vi "Setup Motors.vi"   [LabVIEW 2014]
uses:
  <vilib>/Rock Robotics/SystemInterfaces/DIO/FPGA_DIOPWMChannel.ctl
  <vilib>/Rock Robotics/SystemInterfaces/Typedef/FPGA_TypedefDigitalModule.ctl
  <vilib>/Rock Robotics/WPI/Joystick/WPI_JoystickDeviceEnum.ctl
  <vilib>/Rock Robotics/SystemInterfaces/Typedef/FPGA_TypedefAnalogModule.ctl
  <vilib>/Rock Robotics/SystemInterfaces/AI/FPGA_AIChannel.ctl
  <vilib>/Rock Robotics/WPI/Solenoid/WPI_SolenoidChannel.ctl
  <vilib>/Rock Robotics/SystemInterfaces/AI/FPGA_AIGyroChannel.ctl
  <vilib>/Rock Robotics/SystemInterfaces/Typedef/FPGA_TypedefAnalogModuleForGyro.ctl
  <vilib>/Rock Robotics/SystemInterfaces/DIO/FPGA_DIOChannel.ctl
  <vilib>/Rock Robotics/WPI/SafetyOutput/WPI_SafetyOutputConfigMenu.ctl
  <vilib>/Rock Robotics/WPI/MotorControl/WPI_MotorControlOpen Talon.vi
  <vilib>/Rock Robotics/WPI/Solenoid/WPI_SolenoidOpenSingle.vi
  <vilib>/Rock Robotics/WPI/Switch/WPI_SwitchOpenLimit.vi
  <vilib>/Rock Robotics/WPI/Counter/WPI_CounterDigitalInputToDigitalSource.vi
  Global Variables.vi
types:
  T1 = typedef "FPGA_DIOChannel.ctl" = enum8{"DIO 0", "DIO 1", "DIO 2", "DIO 3", "DIO 4", "DIO 5", "DIO 6", "DIO 7", "DIO 8", "DIO 9", "DIO MXP 0", "DIO MXP 1", "DIO MXP 2", "DIO MXP 3", "DIO MXP 4", "DIO MXP 5", "DIO MXP 6", "DIO MXP 7", "DIO MXP 8", "DIO MXP 9", "DIO MXP 10", "DIO MXP 11", "DIO MXP 12", "DIO MXP 13", "DIO MXP 14", "DIO MXP 15", "Invalid"}
  T2 = typedef "WPI_SafetyOutputConfigMenu.ctl" = enum16{"Enable", "Disable"}
  T3 = typedef "FPGA_DIOPWMChannel.ctl" = enum8{"PWM 0", "PWM 1", "PWM 2", "PWM 3", "PWM 4", "PWM 5", "PWM 6", "PWM 7", "PWM 8", "PWM 9", "PWM MXP 0", "PWM MXP 1", "PWM MXP 2", "PWM MXP 3", "PWM MXP 4", "PWM MXP 5", "PWM MXP 6", "PWM MXP 7", "PWM MXP 8", "PWM MXP 9", "Invalid"}
  T4 = typedef "FPGA_TypedefDigitalModule.ctl" = enum16{"Controller 1"}
  T5 = typedef "FPGA_TypedefAnalogModuleForGyro.ctl" = enum16{"Controller 1"}
  T6 = typedef "FPGA_AIGyroChannel.ctl" = enum8{"AI 0", "AI 1", "Invalid"}
  T7 = typedef "WPI_SolenoidChannel.ctl" = enum8{"Solenoid 0", "Solenoid 1", "Solenoid 2", "Solenoid 3", "Solenoid 4", "Solenoid 5", "Solenoid 6", "Solenoid 7", "Invalid"}
  T8 = typedef "FPGA_AIChannel.ctl" = enum8{"AI 0", "AI 1", "AI 2", "AI 3", "AI MXP 0", "AI MXP 1", "AI MXP 2", "AI MXP 3", "Invalid"}
  T9 = typedef "FPGA_TypedefAnalogModule.ctl" = enum16{"Controller 1"}
  T10 = typedef "WPI_JoystickDeviceEnum.ctl" = enum16{"USB 0", "USB 1", "USB 2", "USB 3", "USB 4", "USB 5"}
  T11 = typedef "WPI_MotorControlDeviceRef.ctl" = cluster{"DeviceStatus":errorcluster, "Type":T12, "PWM":cluster{"Controller":T4, "PWM Channel":T3, "DeadBand":T13}, "CAN":cluster{"Device Number":u8, "Control Mode":T14, "Semaphore":T15, "Max Vout":dbl, "TalonSRX Control Mode":T16}, "Invert":bool, "TransformRef":T17, "InvTransformRef":T17}
  T12 = typedef "WPI_MotorControlType.ctl" = enum16{"PWM", "CAN", "CANTalonSRX"}
  T13 = typedef "WPI_PWMDeadband.ctl" = cluster{"Name":string, "maxPositivePwm":i32, "minPositivePwm":i32, "centerPwm":i32, "maxNegativePwm":i32, "minNegativePwm":i32, "angularRange":u16}
  T14 = typedef "WPI_CANJaguar_ControlMode.ctl" = enum8{"Percent VBus", "Current", "Speed", "Position", "Voltage"}
  T15 = typedef "Semaphore RefNum" = refnum<k1>
  T16 = typedef "WPI_CANTalonSRX_APIControlMode.ctl" = enum8{"Percent VBus", "Speed", "Position", "Slave", "Unchanged / Invalid"}
  T17 = typedef "WPI_PWMTransform_ConPane.ctl" = refnum<vi>
  T18 = typedef "WPI_GyroDevRef.ctl" = cluster{"DevStatus":errorcluster, "Analog Module":T9, "Analog Channel":T8, "Offset":dbl, "Gain (VoltsPerDegree/Second)":dbl}
  T19 = typedef "WPI_SolenoidDevRef.ctl" = cluster{"DevStatus":errorcluster, "Pneumatics Control Module":u8, "Forward Solenoid Channel":T7, "Reverse Solenoid Channel":T7}
  T20 = typedef "WPI_SwitchDevRef.ctl" = cluster{"DevStatus":errorcluster, "DIO Channel":T1, "Controller":T4, "CntIndex":T21, "Normally Closed":bool}
  T21 = typedef "FPGA_CounterCtrSystemIndex.ctl" = enum8{"Ctr 0", "Ctr 1", "Ctr 2", "Ctr 3", "Ctr 4", "Ctr 5", "Ctr 6", "Ctr 7", "Invalid"}
  T22 = typedef "WPI_DigitalInputDevRef.ctl" = cluster{"DevStatus":errorcluster, "DIO Channel":T1, "Controller":T4}
  T23 = typedef "FPGA_CounterEncoderSourceConvertionLVSourceType.ctl" = cluster{"DevStatus":errorcluster, "AnalogTriggerMode?":bool, "DigitalMode":cluster{"Controller":T4, "DIO Channel":T24}, "AnalogTriggerMode":cluster{"AnalogTriggerIndex":T25, "OutputType":T26}}
  T24 = typedef "FPGA_DIODigitalSourceChannel.ctl" = enum8{"DIO 0", "DIO 1", "DIO 2", "DIO 3", "DIO 4", "DIO 5", "DIO 6", "DIO 7", "DIO 8", "DIO 9", "DIO MXP 0", "DIO MXP 1", "DIO MXP 2", "DIO MXP 3", "DIO MXP 4", "DIO MXP 5", "DIO MXP 6", "DIO MXP 7", "DIO MXP 8", "DIO MXP 9", "DIO MXP 10", "DIO MXP 11", "DIO MXP 12", "DIO MXP 13", "DIO MXP 14", "DIO MXP 15", "Disabled"}
  T25 = typedef "FPGA_AnalogTriggerIndex.ctl" = enum8{"Trig 0", "Trig 1", "Trig 2", "Trig 3", "Trig 4", "Trig 5", "Trig 6", "Trig 7", "Invalid"}
  T26 = typedef "FPGA_AnalogTriggerOutType.ctl" = enum16{"InWindow", "TriggerState", "Rising", "Falling"}
  T27 = typedef "WPI_AnalogChannelDevRef.ctl" = cluster{"DevStatus":errorcluster, "Controller":T9, "Analog Channel":T8}
  T28 = typedef "WPI_EncoderDevRef.ctl" = cluster{"DevStatus":errorcluster, "EncoderIndex":T29, "CounterIndex":T21, "DistancePerCount":dbl, "Decoding Type":T30}
  T29 = typedef "FPGA_EncoderIdx.ctl" = enum8{"Enc 0", "Enc 1", "Enc 2", "Enc 3", "Enc 4", "Enc 5", "Enc 6", "Enc 7", "Invalid"}
  T30 = typedef "WPI_EncoderType.ctl" = enum16{"1x", "2x", "4x"}
  T31 = typedef "WPI_JoystickDevRef.ctl" = cluster{"Device":T10}
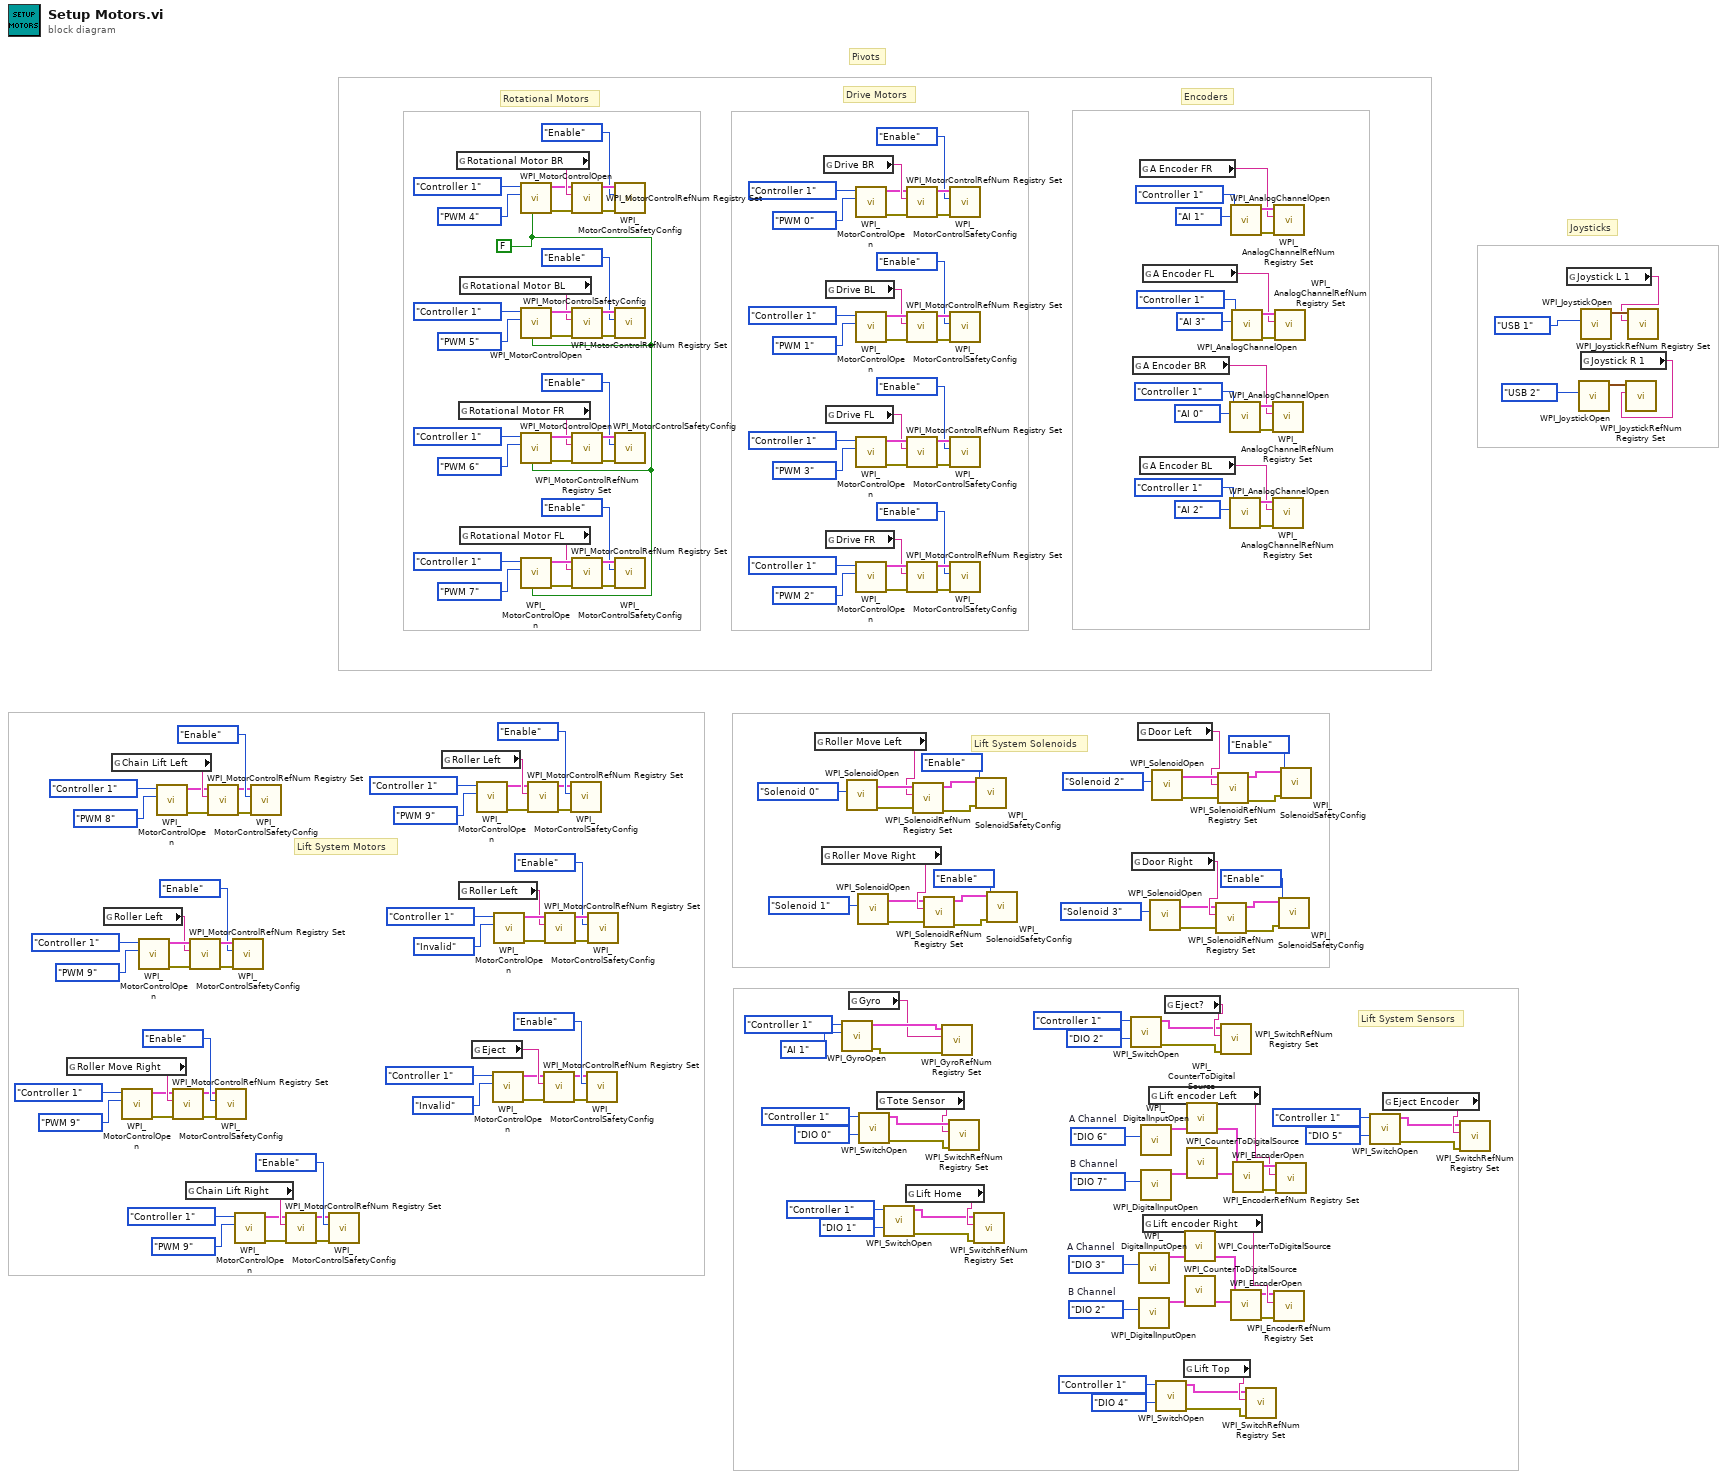
[diagram p0: block diagram]
diagram:
  w1 = FPGA_DIOChannel."DIO 2"  # B Channel
  w2 = FPGA_DIOChannel."DIO 3"  # A Channel
  w18 = FALSE ("Invert")
  w27 = FPGA_DIOChannel."DIO 7"  # B Channel
  w26 = FPGA_DIOChannel."DIO 6"  # A Channel
  # "Lift System Sensors"
  # "Lift System Solenoids"
  # "Lift System Motors"
  # "Encoders"
  # "Joysticks"
  # "Pivots"
  # "Rotational Motors"
  # "Drive Motors"
  n1 = global read "Global Variables.vi" "Roller Move Right"() -> (w116:string)
  n2 = global read "Global Variables.vi" "Roller Left"() -> (w119:string)
  n3 = global read "Global Variables.vi" "Chain Lift Left"() -> (w132:string)
  n4 = call-poly <vilib>:"WPI_MotorControlOpen.vi"("PWM Channel"=FPGA_DIOPWMChannel."PWM 9", "Controller"=FPGA_TypedefDigitalModule."Controller 1") -> ("error out"=w111:errorcluster, "MotorControlDeviceRef"=w110:T11)  [unwired: 8 in]
  n5 = call-poly <vilib>:"WPI_MotorControlOpen.vi"("PWM Channel"=FPGA_DIOPWMChannel."PWM 9", "Controller"=FPGA_TypedefDigitalModule."Controller 1") -> ("error out"=w124:errorcluster, "MotorControlDeviceRef"=w125:T11)  [unwired: 8 in]
  n6 = call-poly <vilib>:"WPI_MotorControlOpen.vi"("PWM Channel"=FPGA_DIOPWMChannel."PWM 8", "Controller"=FPGA_TypedefDigitalModule."Controller 1") -> ("error out"=w127:errorcluster, "MotorControlDeviceRef"=w126:T11)  [unwired: 8 in]
  n7 = call <vilib>:"WPI_MotorControlRefNum Registry Set.vi"("error in (no error)"=w111, "refnum name"=w116, "MotorControlDevRef"=w110) -> ("error out"=w113:errorcluster, "MotorControlDevRef"=w112:T11)  [unwired: 7 in]
  n8 = global read "Global Variables.vi" "Chain Lift Right"() -> (w16:string)
  n9 = call <vilib>:"WPI_MotorControlRefNum Registry Set.vi"("error in (no error)"=w124, "refnum name"=w119, "MotorControlDevRef"=w125) -> ("error out"=w122:errorcluster, "MotorControlDevRef"=w123:T11)  [unwired: 7 in]
  n10 = call <vilib>:"WPI_MotorControlRefNum Registry Set.vi"("error in (no error)"=w127, "refnum name"=w132, "MotorControlDevRef"=w126) -> ("error out"=w129:errorcluster, "MotorControlDevRef"=w128:T11)  [unwired: 7 in]
  n11 = call <vilib>:"WPI_MotorControlSafetyConfig.vi"("error in (no error)"=w113, "mode"=WPI_SafetyOutputConfigMenu."Enable", "MotorControlDevRef"=w112) -> ()  [unwired: 7 in, 2 out]
  n12 = call <vilib>:"WPI_MotorControlSafetyConfig.vi"("error in (no error)"=w122, "mode"=WPI_SafetyOutputConfigMenu."Enable", "MotorControlDevRef"=w123) -> ()  [unwired: 7 in, 2 out]
  n13 = call-poly <vilib>:"WPI_MotorControlOpen.vi"("PWM Channel"=FPGA_DIOPWMChannel."PWM 9", "Controller"=FPGA_TypedefDigitalModule."Controller 1") -> ("error out"=w11:errorcluster, "MotorControlDeviceRef"=w10:T11)  [unwired: 8 in]
  n14 = call <vilib>:"WPI_MotorControlSafetyConfig.vi"("error in (no error)"=w129, "mode"=WPI_SafetyOutputConfigMenu."Enable", "MotorControlDevRef"=w128) -> ()  [unwired: 7 in, 2 out]
  n15 = call <vilib>:"WPI_MotorControlRefNum Registry Set.vi"("error in (no error)"=w11, "refnum name"=w16, "MotorControlDevRef"=w10) -> ("error out"=w13:errorcluster, "MotorControlDevRef"=w12:T11)  [unwired: 7 in]
  n16 = call <vilib>:"WPI_MotorControlSafetyConfig.vi"("error in (no error)"=w13, "mode"=WPI_SafetyOutputConfigMenu."Enable", "MotorControlDevRef"=w12) -> ()  [unwired: 7 in, 2 out]
  n17 = global read "Global Variables.vi" "Roller Left"() -> (w108:string)
  n18 = global read "Global Variables.vi" "Rotational Motor BR"() -> (w186:string)
  n19 = global read "Global Variables.vi" "Rotational Motor FR"() -> (w160:string)
  n20 = global read "Global Variables.vi" "Roller Left"() -> (w95:string)
  n21 = global read "Global Variables.vi" "Rotational Motor BL"() -> (w161:string)
  n22 = global read "Global Variables.vi" "Rotational Motor FL"() -> (w159:string)
  n23 = global read "Global Variables.vi" "Eject"() -> (w92:string)
  n24 = call-poly <vilib>:"WPI_MotorControlOpen.vi"("PWM Channel"=FPGA_DIOPWMChannel."PWM 9", "Controller"=FPGA_TypedefDigitalModule."Controller 1") -> ("error out"=w103:errorcluster, "MotorControlDeviceRef"=w102:T11)  [unwired: 8 in]
  n25 = call-poly <vilib>:"WPI_MotorControlOpen.vi"("PWM Channel"=FPGA_DIOPWMChannel."Invalid", "Controller"=FPGA_TypedefDigitalModule."Controller 1") -> ("error out"=w87:errorcluster, "MotorControlDeviceRef"=w86:T11)  [unwired: 8 in]
  n26 = call-poly <vilib>:"WPI_MotorControlOpen.vi"("PWM Channel"=FPGA_DIOPWMChannel."Invalid", "Controller"=FPGA_TypedefDigitalModule."Controller 1") -> ("error out"=w100:errorcluster, "MotorControlDeviceRef"=w101:T11)  [unwired: 8 in]
  n27 = call-poly <vilib>:"WPI_MotorControlOpen.vi"("Invert"=w18, "PWM Channel"=FPGA_DIOPWMChannel."PWM 4", "Controller"=FPGA_TypedefDigitalModule."Controller 1") -> ("error out"=w184:errorcluster, "MotorControlDeviceRef"=w185:T11)  [unwired: 7 in]
  n28 = call-poly <vilib>:"WPI_MotorControlOpen.vi"("Invert"=w18, "PWM Channel"=FPGA_DIOPWMChannel."PWM 5", "Controller"=FPGA_TypedefDigitalModule."Controller 1") -> ("error out"=w178:errorcluster, "MotorControlDeviceRef"=w179:T11)  [unwired: 7 in]
  n29 = call-poly <vilib>:"WPI_MotorControlOpen.vi"("Invert"=w18, "PWM Channel"=FPGA_DIOPWMChannel."PWM 6", "Controller"=FPGA_TypedefDigitalModule."Controller 1") -> ("error out"=w172:errorcluster, "MotorControlDeviceRef"=w173:T11)  [unwired: 7 in]
  n30 = call-poly <vilib>:"WPI_MotorControlOpen.vi"("Invert"=w18, "PWM Channel"=FPGA_DIOPWMChannel."PWM 7", "Controller"=FPGA_TypedefDigitalModule."Controller 1") -> ("error out"=w166:errorcluster, "MotorControlDeviceRef"=w167:T11)  [unwired: 7 in]
  n31 = call <vilib>:"WPI_MotorControlRefNum Registry Set.vi"("error in (no error)"=w103, "refnum name"=w108, "MotorControlDevRef"=w102) -> ("error out"=w105:errorcluster, "MotorControlDevRef"=w104:T11)  [unwired: 7 in]
  n32 = call <vilib>:"WPI_MotorControlRefNum Registry Set.vi"("error in (no error)"=w87, "refnum name"=w92, "MotorControlDevRef"=w86) -> ("error out"=w89:errorcluster, "MotorControlDevRef"=w88:T11)  [unwired: 7 in]
  n33 = call <vilib>:"WPI_MotorControlRefNum Registry Set.vi"("error in (no error)"=w100, "refnum name"=w95, "MotorControlDevRef"=w101) -> ("error out"=w98:errorcluster, "MotorControlDevRef"=w99:T11)  [unwired: 7 in]
  n34 = call <vilib>:"WPI_MotorControlSafetyConfig.vi"("error in (no error)"=w105, "mode"=WPI_SafetyOutputConfigMenu."Enable", "MotorControlDevRef"=w104) -> ()  [unwired: 7 in, 2 out]
  n35 = call <vilib>:"WPI_MotorControlRefNum Registry Set.vi"("error in (no error)"=w184, "refnum name"=w186, "MotorControlDevRef"=w185) -> ("error out"=w182:errorcluster, "MotorControlDevRef"=w183:T11)  [unwired: 7 in]
  n36 = call <vilib>:"WPI_MotorControlRefNum Registry Set.vi"("error in (no error)"=w178, "refnum name"=w161, "MotorControlDevRef"=w179) -> ("error out"=w176:errorcluster, "MotorControlDevRef"=w177:T11)  [unwired: 7 in]
  n37 = call <vilib>:"WPI_MotorControlRefNum Registry Set.vi"("error in (no error)"=w172, "refnum name"=w160, "MotorControlDevRef"=w173) -> ("error out"=w170:errorcluster, "MotorControlDevRef"=w171:T11)  [unwired: 7 in]
  n38 = call <vilib>:"WPI_MotorControlRefNum Registry Set.vi"("error in (no error)"=w166, "refnum name"=w159, "MotorControlDevRef"=w167) -> ("error out"=w164:errorcluster, "MotorControlDevRef"=w165:T11)  [unwired: 7 in]
  n39 = call <vilib>:"WPI_MotorControlSafetyConfig.vi"("error in (no error)"=w89, "mode"=WPI_SafetyOutputConfigMenu."Enable", "MotorControlDevRef"=w88) -> ()  [unwired: 7 in, 2 out]
  n40 = call <vilib>:"WPI_MotorControlSafetyConfig.vi"("error in (no error)"=w98, "mode"=WPI_SafetyOutputConfigMenu."Enable", "MotorControlDevRef"=w99) -> ()  [unwired: 7 in, 2 out]
  n41 = call <vilib>:"WPI_MotorControlSafetyConfig.vi"("error in (no error)"=w182, "mode"=WPI_SafetyOutputConfigMenu."Enable", "MotorControlDevRef"=w183) -> ()  [unwired: 7 in, 2 out]
  n42 = call <vilib>:"WPI_MotorControlSafetyConfig.vi"("error in (no error)"=w176, "mode"=WPI_SafetyOutputConfigMenu."Enable", "MotorControlDevRef"=w177) -> ()  [unwired: 7 in, 2 out]
  n43 = call <vilib>:"WPI_MotorControlSafetyConfig.vi"("error in (no error)"=w170, "mode"=WPI_SafetyOutputConfigMenu."Enable", "MotorControlDevRef"=w171) -> ()  [unwired: 7 in, 2 out]
  n44 = call <vilib>:"WPI_MotorControlSafetyConfig.vi"("error in (no error)"=w164, "mode"=WPI_SafetyOutputConfigMenu."Enable", "MotorControlDevRef"=w165) -> ()  [unwired: 7 in, 2 out]
  n45 = global read "Global Variables.vi" "Roller Move Left"() -> (w80:string)
  n46 = global read "Global Variables.vi" "Roller Move Right"() -> (w79:string)
  n47 = global read "Global Variables.vi" "Drive BR"() -> (w223:string)
  n48 = global read "Global Variables.vi" "Drive BL"() -> (w198:string)
  n49 = global read "Global Variables.vi" "Drive FL"() -> (w197:string)
  n50 = global read "Global Variables.vi" "Drive FR"() -> (w196:string)
  n51 = call <vilib>:"WPI_GyroOpen.vi"("Analog Channel"=FPGA_AIGyroChannel."AI 1", "Controller"=FPGA_TypedefAnalogModuleForGyro."Controller 1") -> ("error out"=w60:errorcluster, "GyroDevRef"=w61:T18)  [unwired: 7 in, 1 out]
  n52 = call-poly <vilib>:"WPI_SolenoidOpen.vi"("Solenoid Channel"=WPI_SolenoidChannel."Solenoid 0") -> ("error out"=w82:errorcluster, "SolenoidDevRef"=w83:T19)  [unwired: 9 in]
  n53 = global read "Global Variables.vi" "Gyro"() -> (w57:string)
  n54 = call-poly <vilib>:"WPI_MotorControlOpen.vi"("PWM Channel"=FPGA_DIOPWMChannel."PWM 0", "Controller"=FPGA_TypedefDigitalModule."Controller 1") -> ("error out"=w221:errorcluster, "MotorControlDeviceRef"=w222:T11)  [unwired: 8 in]
  n55 = call-poly <vilib>:"WPI_MotorControlOpen.vi"("PWM Channel"=FPGA_DIOPWMChannel."PWM 1", "Controller"=FPGA_TypedefDigitalModule."Controller 1") -> ("error out"=w215:errorcluster, "MotorControlDeviceRef"=w216:T11)  [unwired: 8 in]
  n56 = call-poly <vilib>:"WPI_MotorControlOpen.vi"("PWM Channel"=FPGA_DIOPWMChannel."PWM 3", "Controller"=FPGA_TypedefDigitalModule."Controller 1") -> ("error out"=w209:errorcluster, "MotorControlDeviceRef"=w210:T11)  [unwired: 8 in]
  n57 = call-poly <vilib>:"WPI_MotorControlOpen.vi"("PWM Channel"=FPGA_DIOPWMChannel."PWM 2", "Controller"=FPGA_TypedefDigitalModule."Controller 1") -> ("error out"=w203:errorcluster, "MotorControlDeviceRef"=w204:T11)  [unwired: 8 in]
  n58 = call-poly <vilib>:"WPI_SolenoidOpen.vi"("Solenoid Channel"=WPI_SolenoidChannel."Solenoid 1") -> ("error out"=w77:errorcluster, "SolenoidDevRef"=w76:T19)  [unwired: 9 in]
  n59 = call-poly <vilib>:"WPI_SwitchOpen.vi"("DIO Channel"=FPGA_DIOChannel."DIO 0", "Controller"=FPGA_TypedefDigitalModule."Controller 1") -> ("error out"=w55:errorcluster, "SwitchDevRef"=w56:T20)  [unwired: 8 in]
  n60 = global read "Global Variables.vi" "Tote Sensor"() -> (w52:string)
  n61 = call-poly <vilib>:"WPI_SwitchOpen.vi"("DIO Channel"=FPGA_DIOChannel."DIO 1", "Controller"=FPGA_TypedefDigitalModule."Controller 1") -> ("error out"=w48:errorcluster, "SwitchDevRef"=w47:T20)  [unwired: 8 in]
  n62 = global read "Global Variables.vi" "Lift Home"() -> (w51:string)
  n63 = call <vilib>:"WPI_MotorControlRefNum Registry Set.vi"("error in (no error)"=w221, "refnum name"=w223, "MotorControlDevRef"=w222) -> ("error out"=w219:errorcluster, "MotorControlDevRef"=w220:T11)  [unwired: 7 in]
  n64 = call <vilib>:"WPI_MotorControlRefNum Registry Set.vi"("error in (no error)"=w215, "refnum name"=w198, "MotorControlDevRef"=w216) -> ("error out"=w213:errorcluster, "MotorControlDevRef"=w214:T11)  [unwired: 7 in]
  n65 = call <vilib>:"WPI_MotorControlRefNum Registry Set.vi"("error in (no error)"=w209, "refnum name"=w197, "MotorControlDevRef"=w210) -> ("error out"=w207:errorcluster, "MotorControlDevRef"=w208:T11)  [unwired: 7 in]
  n66 = call <vilib>:"WPI_MotorControlRefNum Registry Set.vi"("error in (no error)"=w203, "refnum name"=w196, "MotorControlDevRef"=w204) -> ("error out"=w201:errorcluster, "MotorControlDevRef"=w202:T11)  [unwired: 7 in]
  n67 = call <vilib>:"WPI_SolenoidRefNum Registry Set.vi"("error in (no error)"=w82, "refnum name"=w80, "SolenoidDevRef"=w83) -> ("error out"=w84:errorcluster, "SolenoidDevRef"=w85:T19)  [unwired: 7 in]
  n68 = call <vilib>:"WPI_SolenoidRefNum Registry Set.vi"("error in (no error)"=w77, "refnum name"=w79, "SolenoidDevRef"=w76) -> ("error out"=w75:errorcluster, "SolenoidDevRef"=w74:T19)  [unwired: 7 in]
  n69 = call <vilib>:"WPI_GyroRefNum Registry Set.vi"("error in (no error)"=w60, "refnum name"=w57, "GyroDevRef"=w61) -> ()  [unwired: 7 in, 2 out]
  n70 = call <vilib>:"WPI_SwitchRefNum Registry Set.vi"("error in (no error)"=w55, "refnum name"=w52, "SwitchDevRef"=w56) -> ()  [unwired: 7 in, 2 out]
  n71 = call <vilib>:"WPI_MotorControlSafetyConfig.vi"("error in (no error)"=w219, "mode"=WPI_SafetyOutputConfigMenu."Enable", "MotorControlDevRef"=w220) -> ()  [unwired: 7 in, 2 out]
  n72 = call <vilib>:"WPI_MotorControlSafetyConfig.vi"("error in (no error)"=w213, "mode"=WPI_SafetyOutputConfigMenu."Enable", "MotorControlDevRef"=w214) -> ()  [unwired: 7 in, 2 out]
  n73 = call <vilib>:"WPI_MotorControlSafetyConfig.vi"("error in (no error)"=w207, "mode"=WPI_SafetyOutputConfigMenu."Enable", "MotorControlDevRef"=w208) -> ()  [unwired: 7 in, 2 out]
  n74 = call <vilib>:"WPI_MotorControlSafetyConfig.vi"("error in (no error)"=w201, "mode"=WPI_SafetyOutputConfigMenu."Enable", "MotorControlDevRef"=w202) -> ()  [unwired: 7 in, 2 out]
  n75 = call <vilib>:"WPI_SwitchRefNum Registry Set.vi"("error in (no error)"=w48, "refnum name"=w51, "SwitchDevRef"=w47) -> ()  [unwired: 7 in, 2 out]
  n76 = call <vilib>:"WPI_SolenoidSafetyConfig.vi"("error in (no error)"=w84, "mode"=WPI_SafetyOutputConfigMenu."Enable", "SolenoidDevRef"=w85) -> ()  [unwired: 7 in, 2 out]
  n77 = call <vilib>:"WPI_SolenoidSafetyConfig.vi"("error in (no error)"=w75, "mode"=WPI_SafetyOutputConfigMenu."Enable", "SolenoidDevRef"=w74) -> ()  [unwired: 7 in, 2 out]
  n78 = call-poly <vilib>:"WPI_SwitchOpen.vi"("DIO Channel"=FPGA_DIOChannel."DIO 2", "Controller"=FPGA_TypedefDigitalModule."Controller 1") -> ("error out"=w38:errorcluster, "SwitchDevRef"=w37:T20)  [unwired: 8 in]
  n79 = global read "Global Variables.vi" "Door Right"() -> (w67:string)
  n80 = global read "Global Variables.vi" "A Encoder BR"() -> (w135:string)
  n81 = global read "Global Variables.vi" "Door Left"() -> (w68:string)
  n82 = call <vilib>:"WPI_DigitalInputOpen.vi"("DIO Channel"=w2) -> ("DigitalInputDevRef"=w5:T22)  [unwired: 2 in, 8 out]
  n83 = call <vilib>:"WPI_DigitalInputOpen.vi"("DIO Channel"=w1) -> ("DigitalInputDevRef"=w4:T22)  [unwired: 2 in, 8 out]
  n84 = global read "Global Variables.vi" "A Encoder FR"() -> (w137:string)
  n85 = global read "Global Variables.vi" "A Encoder BL"() -> (w136:string)
  n86 = call <vilib>:"WPI_DigitalInputOpen.vi"("DIO Channel"=w26) -> ("DigitalInputDevRef"=w23:T22)  [unwired: 2 in, 8 out]
  n87 = call <vilib>:"WPI_DigitalInputOpen.vi"("DIO Channel"=w27) -> ("DigitalInputDevRef"=w24:T22)  [unwired: 2 in, 8 out]
  n88 = global read "Global Variables.vi" "A Encoder FL"() -> (w134:string)
  n89 = global read "Global Variables.vi" "Lift encoder Right"() -> (w9:string)
  n90 = global read "Global Variables.vi" "Lift encoder Left"() -> (w19:string)
  n91 = call-poly <vilib>:"WPI_SolenoidOpen.vi"("Solenoid Channel"=WPI_SolenoidChannel."Solenoid 3") -> ("error out"=w65:errorcluster, "SolenoidDevRef"=w64:T19)  [unwired: 9 in]
  n92 = call-poly <vilib>:"WPI_SolenoidOpen.vi"("Solenoid Channel"=WPI_SolenoidChannel."Solenoid 2") -> ("error out"=w70:errorcluster, "SolenoidDevRef"=w71:T19)  [unwired: 9 in]
  n93 = call-poly <vilib>:"WPI_SwitchOpen.vi"("DIO Channel"=FPGA_DIOChannel."DIO 4", "Controller"=FPGA_TypedefDigitalModule."Controller 1") -> ("error out"=w43:errorcluster, "SwitchDevRef"=w42:T20)  [unwired: 8 in]
  n94 = global read "Global Variables.vi" "Eject?"() -> (w41:string)
  n95 = global read "Global Variables.vi" "Lift Top"() -> (w46:string)
  n96 = call-poly <vilib>:"WPI_CounterToDigitalSource.vi"("DigitalInputDevRef"=w5) -> ("Digital Source"=w6:T23)  [unwired: 6 out]
  n97 = call-poly <vilib>:"WPI_CounterToDigitalSource.vi"("DigitalInputDevRef"=w4) -> ("Digital Source"=w3:T23)  [unwired: 6 out]
  n98 = call-poly <vilib>:"WPI_CounterToDigitalSource.vi"("DigitalInputDevRef"=w23) -> ("Digital Source"=w22:T23)  [unwired: 6 out]
  n99 = call-poly <vilib>:"WPI_CounterToDigitalSource.vi"("DigitalInputDevRef"=w24) -> ("Digital Source"=w25:T23)  [unwired: 6 out]
  n100 = call <vilib>:"WPI_SolenoidRefNum Registry Set.vi"("error in (no error)"=w65, "refnum name"=w67, "SolenoidDevRef"=w64) -> ("error out"=w63:errorcluster, "SolenoidDevRef"=w62:T19)  [unwired: 7 in]
  n101 = call <vilib>:"WPI_SolenoidRefNum Registry Set.vi"("error in (no error)"=w70, "refnum name"=w68, "SolenoidDevRef"=w71) -> ("error out"=w72:errorcluster, "SolenoidDevRef"=w73:T19)  [unwired: 7 in]
  n102 = call <vilib>:"WPI_SwitchRefNum Registry Set.vi"("error in (no error)"=w38, "refnum name"=w41, "SwitchDevRef"=w37) -> ()  [unwired: 7 in, 2 out]
  n103 = call <vilib>:"WPI_AnalogChannelOpen.vi"("Analog Channel"=FPGA_AIChannel."AI 0", "Controller"=FPGA_TypedefAnalogModule."Controller 1") -> ("error out"=w144:errorcluster, "AIDeviceRef"=w145:T27)  [unwired: 8 in]
  n104 = call <vilib>:"WPI_AnalogChannelOpen.vi"("Analog Channel"=FPGA_AIChannel."AI 2", "Controller"=FPGA_TypedefAnalogModule."Controller 1") -> ("error out"=w140:errorcluster, "AIDeviceRef"=w141:T27)  [unwired: 8 in]
  n105 = call <vilib>:"WPI_AnalogChannelOpen.vi"("Analog Channel"=FPGA_AIChannel."AI 1", "Controller"=FPGA_TypedefAnalogModule."Controller 1") -> ("error out"=w152:errorcluster, "AIDeviceRef"=w153:T27)  [unwired: 8 in]
  n106 = call <vilib>:"WPI_EncoderOpen.vi"("BSource"=w3, "ASource"=w6) -> ("error out"=w7:errorcluster, "EncoderDevRef"=w8:T28)  [unwired: 6 in, 2 out]
  n107 = call <vilib>:"WPI_AnalogChannelOpen.vi"("Analog Channel"=FPGA_AIChannel."AI 3", "Controller"=FPGA_TypedefAnalogModule."Controller 1") -> ("error out"=w148:errorcluster, "AIDeviceRef"=w149:T27)  [unwired: 8 in]
  n108 = call <vilib>:"WPI_EncoderOpen.vi"("BSource"=w25, "ASource"=w22) -> ("error out"=w21:errorcluster, "EncoderDevRef"=w20:T28)  [unwired: 6 in, 2 out]
  n109 = call <vilib>:"WPI_SwitchRefNum Registry Set.vi"("error in (no error)"=w43, "refnum name"=w46, "SwitchDevRef"=w42) -> ()  [unwired: 7 in, 2 out]
  n110 = call <vilib>:"WPI_AnalogChannelRefNum Registry Set.vi"("error in (no error)"=w144, "refnum name"=w135, "AIDeviceRef"=w145) -> ()  [unwired: 7 in, 2 out]
  n111 = call <vilib>:"WPI_AnalogChannelRefNum Registry Set.vi"("error in (no error)"=w140, "refnum name"=w136, "AIDeviceRef"=w141) -> ()  [unwired: 7 in, 2 out]
  n112 = call <vilib>:"WPI_AnalogChannelRefNum Registry Set.vi"("error in (no error)"=w152, "refnum name"=w137, "AIDeviceRef"=w153) -> ()  [unwired: 7 in, 2 out]
  n113 = call <vilib>:"WPI_EncoderRefNum Registry Set.vi"("error in (no error)"=w7, "refnum name"=w9, "EncoderDevRef"=w8) -> ()  [unwired: 7 in, 2 out]
  n114 = call <vilib>:"WPI_AnalogChannelRefNum Registry Set.vi"("error in (no error)"=w148, "refnum name"=w134, "AIDeviceRef"=w149) -> ()  [unwired: 7 in, 2 out]
  n115 = call <vilib>:"WPI_EncoderRefNum Registry Set.vi"("error in (no error)"=w21, "refnum name"=w19, "EncoderDevRef"=w20) -> ()  [unwired: 7 in, 2 out]
  n116 = call <vilib>:"WPI_SolenoidSafetyConfig.vi"("error in (no error)"=w63, "mode"=WPI_SafetyOutputConfigMenu."Enable", "SolenoidDevRef"=w62) -> ()  [unwired: 7 in, 2 out]
  n117 = call <vilib>:"WPI_SolenoidSafetyConfig.vi"("error in (no error)"=w72, "mode"=WPI_SafetyOutputConfigMenu."Enable", "SolenoidDevRef"=w73) -> ()  [unwired: 7 in, 2 out]
  n118 = call-poly <vilib>:"WPI_SwitchOpen.vi"("DIO Channel"=FPGA_DIOChannel."DIO 5", "Controller"=FPGA_TypedefDigitalModule."Controller 1") -> ("error out"=w33:errorcluster, "SwitchDevRef"=w32:T20)  [unwired: 8 in]
  n119 = global read "Global Variables.vi" "Eject Encoder"() -> (w36:string)
  n120 = call <vilib>:"WPI_SwitchRefNum Registry Set.vi"("error in (no error)"=w33, "refnum name"=w36, "SwitchDevRef"=w32) -> ()  [unwired: 7 in, 2 out]
  n121 = global read "Global Variables.vi" "Joystick L 1"() -> (w190:string)
  n122 = call <vilib>:"WPI_JoystickOpen.vi"("JoystickDevice"=WPI_JoystickDeviceEnum."USB 2") -> ("JoystickDevRef"=w188:T31)  [unwired: 10 in]
  n123 = call <vilib>:"WPI_JoystickOpen.vi"("JoystickDevice"=WPI_JoystickDeviceEnum."USB 1") -> ("JoystickDevRef"=w191:T31)  [unwired: 10 in]
  n124 = global read "Global Variables.vi" "Joystick R 1"() -> (w187:string)
  n125 = call <vilib>:"WPI_JoystickRefNum Registry Set.vi"("refnum name"=w187, "JoystickDevRef"=w188) -> ()  [unwired: 8 in, 2 out]
  n126 = call <vilib>:"WPI_JoystickRefNum Registry Set.vi"("refnum name"=w190, "JoystickDevRef"=w191) -> ()  [unwired: 8 in, 2 out]
